vi "startAutomatedTest.vi"(8 "error in (no error)":errorcluster, 9 "Test Parameters":T1 {"Cycle profile"."Pause After" min=0.0 max=600.0 format="%.1f"; "Cycle profile"."Force Setpoint" min=-888.0 max=888.0 format="%.1f"; "Number of cycles for complete test" min=1}, 10 "model":refnum<class "Model.lvclass">, 11 "InteractiveMotionState in":refnum<class "InteractiveMotionState.lvclass">) -> (0 "error out":errorcluster, 2 "model 2":refnum<class "Model.lvclass">, 3 "InteractiveMotionState out":refnum<class "InteractiveMotionState.lvclass">)   [LabVIEW 2013, in "InteractiveMotionState.lvclass"]
uses:
  InteractiveMotionState.lvclass
  Model/Model/Model.lvclass
  Configuration/Test Parameters.ctl
  Configuration/CycleProfileConfig.ctl
  Typedefs/StateSelector.ctl
  Typedefs/M2AADTTypedefs.lvlib
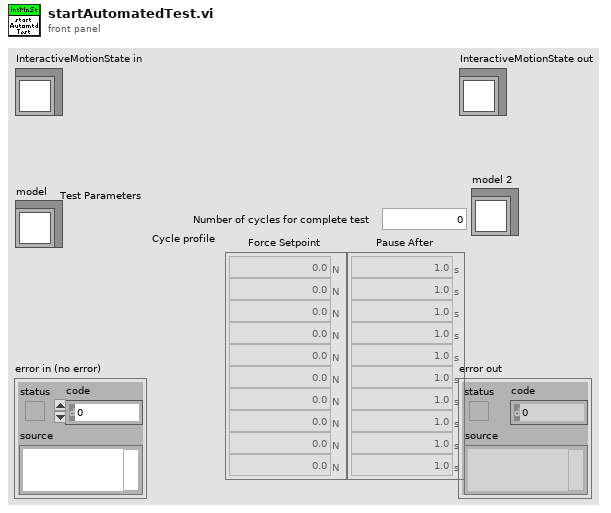
[diagram p1: front panel]
types:
  T1 = typedef "Test Parameters.ctl" = cluster{"Number of cycles for complete test":u32, "Cycle profile":T2}
  T2 = typedef "CycleProfileConfig.ctl" = cluster{"Force Setpoint":dbl[unit][], "Pause After":dbl[unit][]}
  T3 = typedef "M2AADTTypedefs.lvlib/StateSelector.ctl" = enum16{"EndingCycleState", "FaultState", "InteractiveMotionState", "MovingToNewForceState", "OffState", "PausingState", "StandbyState", "StoppedState"}
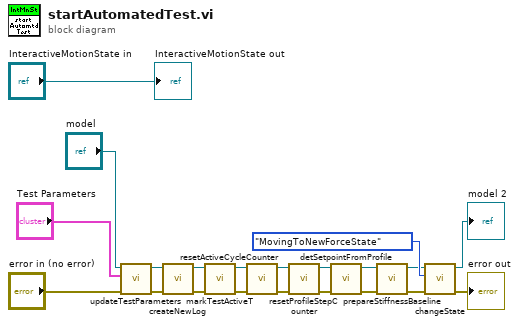
[diagram p0: block diagram]
diagram:
  n1 = call "updateTestParameters.vi"("error in (no error)"="error in (no error)", "Test Parameters"="Test Parameters", "Model in"="model") -> ("error out"=w10:errorcluster, "Model out"=w12:refnum<class "Model.lvclass">)  [unwired: 7 in]
  n2 = call "createNewLog.vi"("error in (no error)"=w10, "Model in"=w12) -> ("error out"=w15:errorcluster, "Model out"=w17:refnum<class "Model.lvclass">)  [unwired: 8 in]
  n3 = call "markTestActiveT.vi"("error in (no error)"=w15, "Model in"=w17) -> ("error out"=w14:errorcluster, "Model out"=w16:refnum<class "Model.lvclass">)  [unwired: 8 in]
  n4 = call "resetActiveCycleCounter.vi"("error in (no error)"=w14, "Model in"=w16) -> ("error out"=w1:errorcluster, "Model out"=w2:refnum<class "Model.lvclass">)  [unwired: 8 in]
  n5 = call "resetProfileStepCounter.vi"("error in (no error)"=w1, "Model in"=w2) -> ("error out"=w7:errorcluster, "Model out"=w8:refnum<class "Model.lvclass">)  [unwired: 8 in]
  n6 = call "detSetpointFromProfile.vi"("error in (no error)"=w7, "Model in"=w8) -> ("error out"=w4:errorcluster, "Model out"=w6:refnum<class "Model.lvclass">)  [unwired: 8 in]
  n7 = call "prepareStiffnessBaseline.vi"("error in (no error)"=w4, "Model in"=w6) -> ("error out"=w3:errorcluster, "Model out"=w5:refnum<class "Model.lvclass">)  [unwired: 8 in]
  n8 = call "changeState.vi"("error in (no error)"=w3, "State:"=StateSelector."MovingToNewForceState", "Model in"=w5) -> ("error out"=→"error out":errorcluster, "Model out"=→"model 2":refnum<class "Model.lvclass">)  [unwired: 7 in]
  "InteractiveMotionState out" <- "InteractiveMotionState in"
